vi "Get Attributes.vi"(8 "error in (no error)":errorcluster, 11 "File in":refnum<class "File.lvclass">) -> (0 "error out":errorcluster, 2 "Attributes":T1, 3 "File out":refnum<class "File.lvclass">)   [LabVIEW 2020, in "File.lvclass"]
uses:
  File.lvclass
  Waveform/Attributes.ctl
  Waveform/Waveform.lvclass
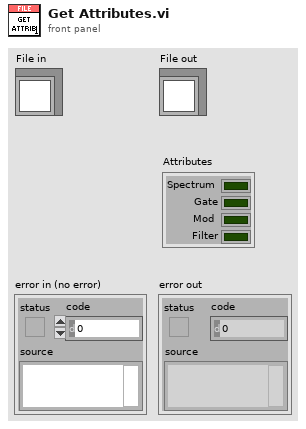
[diagram p1: front panel]
types:
  T1 = typedef "Waveform.lvclass/Attributes.ctl" = cluster{"Spectrum":bool, "Gate":bool, "Mod":bool, "Filter":bool}
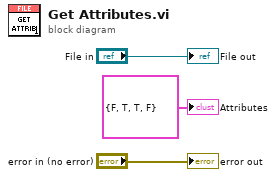
[diagram p0: block diagram]
diagram:
  "error out" <- "error in (no error)"
  "File out" <- "File in"
  "Attributes" <- T1 {"Spectrum"=FALSE, "Gate"=TRUE, "Mod"=TRUE, "Filter"=FALSE} ("Attributes")
